vi "SwerveDriveSetOutputs.vi"(10 "VelocitySetpoints":dbl[](array[numeric]), 11 "AngleSetpoints":dbl[](array[numeric])) -> ()   [LabVIEW 2016]
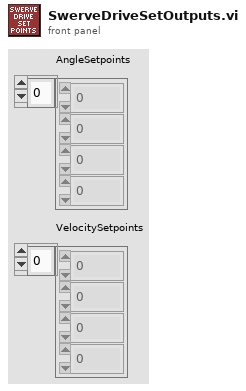
[diagram p1: front panel]
types:
  T1 = typedef "WPI_MotorControlDeviceRef.ctl" = cluster{"DeviceStatus":errorcluster, "Type":T2, "PWM":cluster{"PWM Channel":T3, "DeadBand":T4}, "CAN":cluster{"Device Number":u8, "SetOutput VI Ref":variant, "GetOutput VI Ref":variant, "Enable VI Ref":variant, "Disable VI Ref":variant, "Data":variant}, "Invert":bool}
  T2 = typedef "WPI_MotorControlType.ctl" = enum16{"PWM", "CAN"}
  T3 = typedef "FPGA_DIOPWMChannel.ctl" = enum8{"PWM 0", "PWM 1", "PWM 2", "PWM 3", "PWM 4", "PWM 5", "PWM 6", "PWM 7", "PWM 8", "PWM 9", "PWM MXP 0", "PWM MXP 1", "PWM MXP 2", "PWM MXP 3", "PWM MXP 4", "PWM MXP 5", "PWM MXP 6", "PWM MXP 7", "PWM MXP 8", "PWM MXP 9", "Invalid"}
  T4 = typedef "WPI_PWMDeadband.ctl" = cluster{"Name":string, "maxPositivePwm":i32, "minPositivePwm":i32, "centerPwm":i32, "maxNegativePwm":i32, "minNegativePwm":i32, "angularRange":u16}
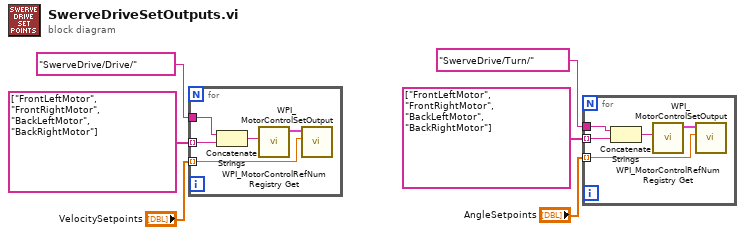
[diagram p0: block diagram]
diagram:
  n1 = for {
    tunnel: "VelocitySetpoints" -> [w11] mode=indexing
    tunnel: string[] ["FrontLeftMotor", "FrontRightMotor", "BackLeftMotor", "BackRightMotor"] -> [w8] mode=indexing
    tunnel: "SwerveDrive/Drive/" ("refnum name") -> [w9]
    n2 = Concatenate Strings(w9, w8) -> (w7:string)
    n3 = call <vilib>:"WPI_MotorControlRefNum Registry Get.vi"("refnum name"=w7) -> ("MotorControlDevRef"=w10:T1)  [unwired: 9 in, 1 out]
    n4 = call <vilib>:"WPI_MotorControlSetOutput.vi"("Output"=w11, "MotorControlDevRef"=w10) -> ()  [unwired: 7 in, 3 out]
  }
  n5 = for {
    tunnel: "AngleSetpoints" -> [w16] mode=indexing
    tunnel: string[] ["FrontLeftMotor", "FrontRightMotor", "BackLeftMotor", "BackRightMotor"] -> [w13] mode=indexing
    tunnel: "SwerveDrive/Turn/" ("refnum name") -> [w14]
    n6 = Concatenate Strings(w14, w13) -> (w12:string)
    n7 = call <vilib>:"WPI_MotorControlRefNum Registry Get.vi"("refnum name"=w12) -> ("MotorControlDevRef"=w15:T1)  [unwired: 9 in, 1 out]
    n8 = call <vilib>:"WPI_MotorControlSetOutput.vi"("Output"=w16, "MotorControlDevRef"=w15) -> ()  [unwired: 7 in, 3 out]
  }
